vi "Shoot.vi"(4 "Icrement Up":bool, 6 "Icrement Down":bool, 9 "Override?":bool, 10 "Shoot?":bool, 11 "Set RPM":dbl=7000.0) -> ()   [LabVIEW 2016]
uses:
  <vilib>/functionblocks/Edge Detection/One Shot Rising with Input/One Shot Rising with Input.vi
  <vilib>/functionblocks/FB Core/FB Core.xnode
  <vilib>/gmath/NI_Gmath.lvlib
  <vilib>/functionblocks/NI_FunctionBlock Libraries.lvlib
panel:
  in  "Increment":dbl format="%#_13g"
  in  "OR Speed":dbl=0.53
  in  "RPM Array":dbl[](array[numeric]) format="%_6g"
  in  "Control":dbl[](array[numeric]) format="%_6g"
  in  "kP":dbl
  out "Shooter RPM":dbl
  out "Shooter RPM":dbl
  out "Encoder Index Count":dbl format="%#_13g"
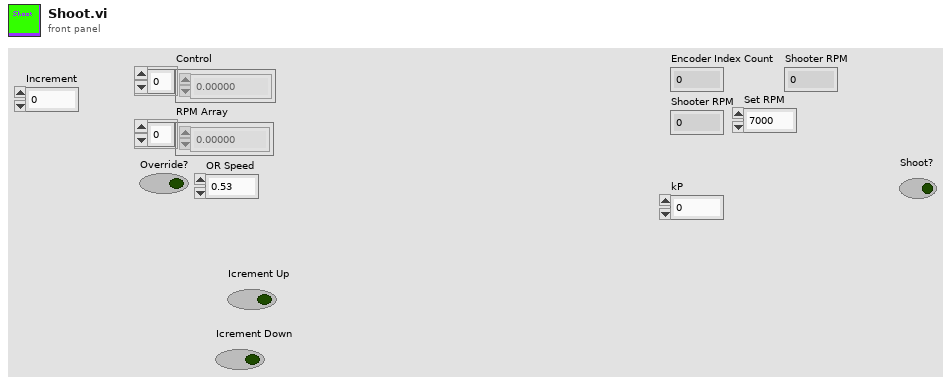
[diagram p1: front panel]
types:
  T1 = typedef "WPI_MotorControlDeviceRef.ctl" = cluster{"DeviceStatus":errorcluster, "Type":T2, "PWM":cluster{"PWM Channel":T3, "DeadBand":T4}, "CAN":cluster{"Device Number":u8, "SetOutput VI Ref":variant, "GetOutput VI Ref":variant, "Enable VI Ref":variant, "Disable VI Ref":variant, "Data":variant}, "Invert":bool}
  T2 = typedef "WPI_MotorControlType.ctl" = enum16{"PWM", "CAN"}
  T3 = typedef "FPGA_DIOPWMChannel.ctl" = enum8{"PWM 0", "PWM 1", "PWM 2", "PWM 3", "PWM 4", "PWM 5", "PWM 6", "PWM 7", "PWM 8", "PWM 9", "PWM MXP 0", "PWM MXP 1", "PWM MXP 2", "PWM MXP 3", "PWM MXP 4", "PWM MXP 5", "PWM MXP 6", "PWM MXP 7", "PWM MXP 8", "PWM MXP 9", "Invalid"}
  T4 = typedef "WPI_PWMDeadband.ctl" = cluster{"Name":string, "maxPositivePwm":i32, "minPositivePwm":i32, "centerPwm":i32, "maxNegativePwm":i32, "minNegativePwm":i32, "angularRange":u16}
  T5 = typedef "WPI_CANTalonSRX_GlobalStatus.ctl" = cluster{"Applied Throttle":dbl, "Module Enabled":bool, "CAN Error":errorcluster, "Closed Loop Error":dbl, "Forward Limit Switch Closed":bool, "Reverse Limit Switch Closed":bool, "Sensor Position":dbl, "Sensor Velocity":dbl, "Current":dbl, "Sticky Fault - Over Temp":bool, "Sticky Fault - Under Voltage":bool, "Sticky Fault - Forward Limit":bool, "Sticky Fault - Reverse Limit":bool, "Sticky Fault - Forward Soft Limit":bool, "Sticky Fault - Reverse Soft Limit":bool, "Brake is Enabled":bool, "Encoder Position":dbl, "Encoder Velocity":dbl, "Encoder Index Count":dbl, "Encoder A Pin State":bool, "Encoder B Pin State":bool, "Encoder Index Pin State":bool, "Analog In":dbl, "Analog In Velocity":dbl, "Temperature (C)":dbl, "Battery Voltage":dbl, "Control 5 Is Supported":bool, "Current Profile Slot Select":dbl, "Pos Div 8":bool, "Vel Div 4":bool, "Pulse Width Position":i32, "Pulse Width Velocity":i32, "Pulse Width Rise To Rise (us)":i32, "Pulse Width Rise To Fall (us)":i32, "Mot Prof Active Is Under Run":bool, "Mot Prof Active Has Under Run":bool, "Mot Prof Active Is Last":bool, "Mot Prof Active Velocity Only":bool, "Mot Prof Active Is Valid":bool, "Mot Prof Buffer Is Full":bool, "Mot Prof Active Profile Slot Select":i32, "Mot Prof NextID":i32, "Mot Prof Count":i32, "Mot Prof Active Velocity":dbl, "Mot Prof Active Position":dbl, "Mot Prof Output Enable":i32}
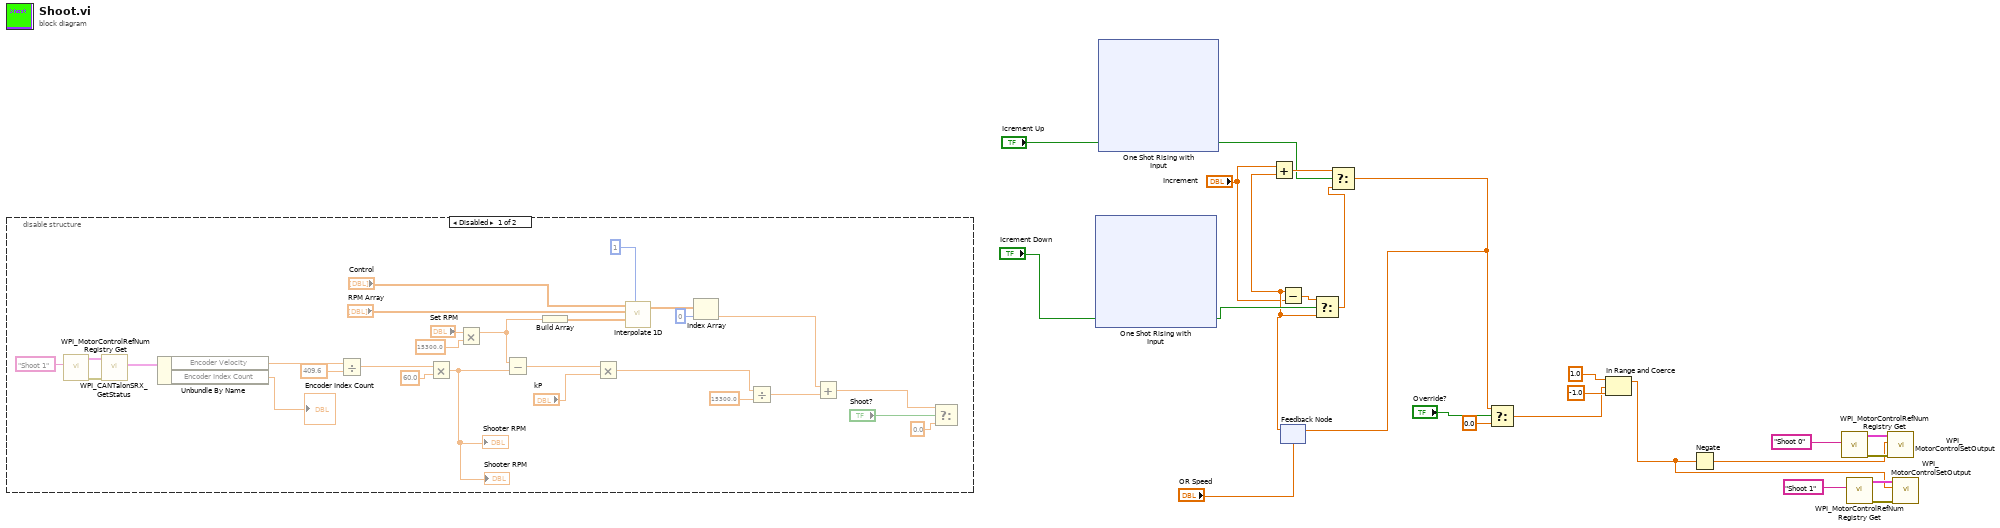
[diagram p0: block diagram]
diagram:
  n1 = disable-structure shown="Disabled" {
    frame Disabled {
      n2 = call <vilib>:"WPI_MotorControlRefNum Registry Get.vi"("refnum name"="Shoot 1") -> ("error out"=w51:errorcluster, "MotorControlDevRef"=w50:T1)  [unwired: 9 in]
      n3 = call <vilib>:"WPI_CANTalonSRX_GetStatus.vi"("error in (no error)"=w51, "CAN Talon SRX Ref"=w50) -> ("Talon SRX Status"=w49:T5)  [unwired: 7 in, 2 out]
      n4 = Unbundle By Name(w49) -> ("Encoder Velocity"=w47:dbl, "Encoder Index Count"=→"Encoder Index Count":dbl)
      n5 = Divide(x=w47, y=409.6) -> (x/y=w45:dbl)
      n6 = Multiply(x=w45, y=60.0) -> (x*y=w43:dbl)
      "Shooter RPM" <- w43
      "Shooter RPM" <- w43
      n7 = Multiply(x="Set RPM", y=15300.0) -> (x*y=w26:dbl)
      n8 = Subtract(x=w26, y=w43) -> (x-y=w39:dbl)
      n9 = Build Array(w26) -> (w37:dbl[])
      n10 = Multiply(x=w39, y="kP") -> (x*y=w33:dbl)
      n11 = call <vilib>:"Interpolate 1D.vi"("method"=1, "xi"=w37, "X"="RPM Array", "Y"="Control") -> ("yi"=w41:dbl[])  [unwired: 5 in, 2 out]
      n12 = Index Array(array=w41, index=0) -> (element=w30:dbl)
      n13 = Divide(x=w33, y=15300.0) -> (x/y=w31:dbl)
      n14 = Add(x=w30, y=w31) -> (x+y=w29:dbl)
      n15 = Select(t=w29, s="Shoot?", f=0.0) -> ()  [unwired: 1 out]
    }
    frame Enabled {
    }
  }
  n16 = xnode "One Shot Rising with Input"("input"="Icrement Down") -> ("output"=w11:bool)  [unwired: 1 in, 1 out]
  n17 = xnode "One Shot Rising with Input"("input"="Icrement Up") -> ("output"=w6:bool)  [unwired: 1 in, 1 out]
  n18 = feedback #1("OR Speed") -> (w2:dbl)
  n19 = Add(x="Increment", y=w2) -> (x+y=w8:dbl)
  n20 = Subtract(x=w2, y="Increment") -> (x-y=w9:dbl)
  n21 = Select(t=w9, s=w11, f=w2) -> (s? t:f=w7:dbl)
  n22 = Select(t=w8, s=w6, f=w7) -> (s? t:f=w4:dbl)
  n23 = feedback-in #1(w4) -> ()
  n24 = Select(t=w4, s="Override?", f=0.0) -> (s? t:f=w3:dbl)
  n25 = In Range and Coerce(upper limit=1.0, x=w3, lower limit=-1.0) -> (coerced(x)=w14:dbl)  [unwired: 1 out]
  n26 = Negate(x=w14) -> (-x=w15:dbl)
  n27 = call <vilib>:"WPI_MotorControlRefNum Registry Get.vi"("refnum name"="Shoot 0") -> ("error out"=w22:errorcluster, "MotorControlDevRef"=w20:T1)  [unwired: 9 in]
  n28 = call <vilib>:"WPI_MotorControlRefNum Registry Get.vi"("refnum name"="Shoot 1") -> ("error out"=w19:errorcluster, "MotorControlDevRef"=w23:T1)  [unwired: 9 in]
  n29 = call <vilib>:"WPI_MotorControlSetOutput.vi"("error in (no error)"=w22, "Output"=w15, "MotorControlDevRef"=w20) -> ()  [unwired: 6 in, 3 out]
  n30 = call <vilib>:"WPI_MotorControlSetOutput.vi"("error in (no error)"=w19, "Output"=w14, "MotorControlDevRef"=w23) -> ()  [unwired: 6 in, 3 out]
